vi "1big_with_d12.vi"() -> ()   [LabVIEW 2021]
panel:
  out "Waveform Graph":dbl[](graph)=[0.0, 0.0048018876, 0.018431017, 0.039760882, 0.067719858, 0.10129508, 0.13953534, 0.18155307, 0.2265255, 0.27369508, 0.32236922, 0.37191952, 0.42178034, 0.47144713, 0.52047418, 0.56847222, 0.61510569, 0.66008982, 0.70318758, 0.74420648, 0.78299539, 0.81944126, 0.8534659, 0.88502272, 0.91409368, 0.94068615, 0.96483002, 0.98657486, 1.0059872, 1.023148, 1.0381504, 1.0510971, 1.0620986, 1.0712715, 1.078736, 1.0846151, 1.0890327, 1.0921125, 1.0939767, 1.0947453, 1.0945349, 1.0934583, 1.0916234, 1.0891333, 1.0860856, 1.082572, 1.0786782, 1.074484, 1.0700627, 1.0654817, 1.0608022, 1.0560794, 1.0513626, 1.0466956, 1.0421167, 1.037659, 1.0333508, 1.0292157, 1.0252732, 1.0215385, 1.0180234, 1.014736, 1.0116817, 1.0088627, 1.006279, 1.0039284, 1.0018066, 0.99990777, 0.99822449, 0.99674827, 0.9954696, 0.99437817, 0.9934631, 0.99271305, 0.99211642, 0.99166149, 0.99133651, 0.99112985, 0.99103008, 0.99102605, 0.99110696, 0.99126246, 0.99148264, 0.99175812, 0.99208005, 0.99244014, 0.9928307, 0.99324459, 0.99367528, 0.99411683, 0.99456383, 0.99501148, 0.99545547, 0.99589204, 0.99631793, 0.99673032, 0.99712687, 0.99750563, 0.99786504, 0.99820391, 0.99852138, 0.99881687, 0.99909008, 0.99934096, 0.99956969, 0.99977659, 0.99996221, 1.0001272, 1.0002723, 1.0003985, 1.0005066, 1.0005977, 1.000673, 1.0007333, 1.0007799, 1.000814, 1.0008365, 1.0008486, 1.0008513, 1.0008457, 1.0008328, 1.0008135, 1.0007887, 1.0007593, 1.0007261, 1.0006897, 1.000651, 1.0006106, 1.000569, 1.0005267, 1.0004842, 1.000442, 1.0004004, 1.0003598, 1.0003203, 1.0002823, 1.0002459, 1.0002114, 1.0001787, 1.0001481, 1.0001195, 1.000093, 1.0000687, 1.0000464, 1.0000263, 1.0000081, 0.99999198, 0.99997772, 0.99996529, 0.99995459, 0.99994552, 0.999938, 0.99993191, 0.99992715, 0.99992361, 0.99992119, 0.99991979, 0.9999193, 0.99991963, 0.99992068, 0.99992235, 0.99992457, 0.99992724, 0.9999303, 0.99993367, 0.99993728, 0.99994108, 0.999945, 0.99994899, 0.99995302, 0.99995703, 0.99996099, 0.99996487, 0.99996864, 0.99997229, 0.99997578, 0.9999791, 0.99998225, 0.9999852, 0.99998796, 0.99999053, 0.99999289, 0.99999505, 0.99999701, 0.99999878, 1.0000004, 1.0000018, 1.000003, 1.000004, 1.0000049, 1.0000057, 1.0000063, 1.0000068, 1.0000072, 1.0000074, 1.0000076, 1.0000076, 1.0000076, 1.0000076, 1.0000074, 1.0000072]
  out "size(s)":i32[](array[numeric])=[603, 2]
  out "Signals 2":dbl=1.0000072
  out "Signals":dynamicdata(graph)=[{"t0"=timestamp(0 s since 1904-01-01), "dt"=1.0, "Y"=array[603 elements], "attributes"=variant("NI_ChannelName"=variant(string ""), "NI_ExpIsRelativeTime"=variant(bool FALSE), "NI_ExpStartTimeStamp"=variant(timestamp timestamp(0 s since 1904-01-01)), "NI_ExpTimeStamp"=variant(timestamp timestamp(0 s since 1904-01-01)), "NI_ExpXDimension"=variant(string ""))}, {"t0"=timestamp(0 s since 1904-01-01), "dt"=1.0, "Y"=[0.0, 0.0, 0.0, 0.0, 0.0, 0.0, 0.0, 0.0, 0.0, 0.0, 0.0, 0.0, 0.0, 0.0, 0.0, 0.0, 0.0, 0.0, 0.0, 0.0, 0.0, 0.0, 0.0, 0.0, 0.0, 0.0, 0.0, 0.0, 0.0, 0.0, 0.0, 0.0, 0.0, 0.0, 0.0, 0.0, 0.0, 0.0, 0.0, 0.0, 0.0, 0.0, 0.0, 0.0, 0.0, 0.0, 0.0, 0.0, 0.0, 0.0, 0.0, 0.0, 0.0, 0.0, 0.0, 0.0, 0.0, 0.0, 0.0, 0.0, 0.0, 0.0, 0.0, 0.0, 0.0, 0.0, 0.0, 0.0, 0.0, 0.0, 0.0, 0.0, 0.0, 0.0, 0.0, 0.0, 0.0, 0.0, 0.0, 0.0, 0.0, 0.0, 0.0, 0.0, 0.0, 0.0, 0.0, 0.0, 0.0, 0.0, 0.0, 0.0, 0.0, 0.0, 0.0, 0.0, 0.0, 0.0, 0.0, 0.0, 0.0, 0.0, 0.0, 0.0, 0.0, 0.0, 0.0, 0.0, 0.0, 0.0, 0.0, 0.0, 0.0, 0.0, 0.0, 0.0, 0.0, 0.0, 0.0, 0.0, 0.0, 0.0, 0.0, 0.0, 0.0, 0.0, 0.0, 0.0, 0.0, 0.0, 0.0, 0.0, 0.0, 0.0, 0.0, 0.0, 0.0, 0.0, 0.0, 0.0, 0.0, 0.0, 0.0, 0.0, 0.0, 0.0, 0.0, 0.0, 0.0, 0.0, 0.0, 0.0, 0.0, 0.0, 0.0, 0.0, 0.0, 0.0, 0.0, 0.0, 0.0, 0.0, 0.0, 0.0, 0.0, 0.0, 0.0, 0.0, 0.0, 0.0, 0.0, 0.0, 0.0, 0.0, 0.0, 0.0, 0.0, 0.0, 0.0, 0.0, 0.0, 0.0, 0.0, 0.0, 0.0, 0.0, 0.0, 0.0, 0.0, 0.0, 0.0, 0.0, 0.0, 0.0, 0.0, 0.0, 0.0, 0.0, 0.0, 0.0, 0.0, 0.0, 0.0, 0.0, 0.0, 0.0, 0.0, 0.0, 0.0, 0.0, 0.0, 0.0, 0.0, 0.0, 0.0, 0.0, 0.0, 0.0, 0.0, 0.0, 0.0, 0.0, 0.0, 0.0, 0.0, 0.0, 0.0, 0.0, 0.0, 0.0, 0.0, 0.0, 0.0, 0.0, 0.0, 0.0, 0.0, 0.0, 0.0, 0.0, 0.0, 0.0, 0.0, 0.0, 0.0, 0.0, 0.0, 0.0, 0.0, 0.0, 0.0, 0.0, 0.0, 0.0, 0.0, 0.0, 0.0, 0.0, 0.0, 0.0, 0.0, 0.0, 0.0, 0.0, 0.0, 0.0, 0.0, 0.0, 0.0, 0.0, 0.0, 0.0, 0.0, 0.0, 0.0, 0.0, 0.0, 0.0, 0.0, 0.0, 0.0, 0.0, 0.0, 0.0, 0.0, 0.0, 0.0, 0.0, 0.0, 0.0, 0.0, 0.0, 0.0, 0.0, 0.0, 0.0, 0.0, 0.0, 0.0, 0.0, 0.0, 0.0, 0.0, 0.0, 0.0, 0.0, 0.0, 0.0, 0.0, 0.0, 0.0, 0.0, 0.0, 0.0, 0.0, 0.0, 0.0, 0.0, 0.0, 0.0, 0.0, 0.0, 0.0, 0.0, 0.0, 0.0, 0.0, 0.0, 0.0, 0.0, 0.0, 0.0, 0.0, 0.0, 0.0, 0.0, 0.0, 0.0, 0.0, 0.0, 0.0, 0.0, 0.0, 0.0, 0.0, 0.0, 0.0, 0.0, 0.0, 0.0, 0.0, 0.0, 0.0, 0.0, 0.0, 0.0, 0.0, 0.0, 0.0, 0.0, 0.0, 0.0, 0.0, 0.0, 0.0, 0.0, 0.0, 0.0, 0.0, 0.0, 0.0, 0.0, 0.0, 0.0, 0.0, 0.0, 0.0, 0.0, 0.0, 0.0, 0.0, 0.0, 0.0, 0.0, 0.0, 0.0, 0.0, 0.0, 0.0, 0.0, 0.0, 0.0, 0.0, 0.0, 0.0, 0.0, 0.0, 0.0, 0.0, 0.0, 0.0, 0.0, 0.0, 0.0, 0.0, 0.0, 0.0, 0.0, 0.0, 0.0, 0.0, 0.0, 0.0, 0.0, 0.0, 0.0, 0.0, 0.0, 0.0, 0.0, 0.0, 0.0, 0.0, 0.0, 0.0, 0.0, 0.0, 0.0, 0.0, 0.0, 0.0, 0.0, 0.0, 0.0, 0.0, 0.0, 0.0, 0.0, 0.0, 0.0, 0.0, 0.0, 0.0, 0.0, 0.0, 0.0, 0.0, 0.0, 0.0, 0.0, 0.0, 0.0, 0.0, 0.0, 0.0, 0.0, 0.0, 0.0, 0.0, 0.0, 0.0, 0.0, 0.0, 0.0, 0.0, 0.0, 0.0, 0.0, 0.0, 0.0, 0.0, 0.0, 0.0, 0.0, 0.0, 0.0, 0.0, 0.0, 0.0, 0.0, 0.0, 0.0, 0.0, 0.0, 0.0, 0.0, 0.0, 0.0, 0.0, 0.0, 0.0, 0.0, 0.0, 0.0, 0.0, 0.0, 0.0, 0.0, 0.0, 0.0, 0.0, 0.0, 0.0, 0.0, 0.0, 0.0, 0.0, 0.0, 0.0, 0.0, 0.0, 0.0, 0.0, 0.0, 0.0, 0.0, 0.0, 0.0, 0.0, 0.0, 0.0, 0.0, 0.0, 0.0, 0.0, 0.0, 0.0, 0.0, 0.0, 0.0, 0.0, 0.0, 0.0, 0.0, 0.0, 0.0, 0.0, 0.0, 0.0, 0.0, 0.0, 0.0, 0.0, 0.0, 0.0, 0.0, 0.0, 0.0, 0.0, 0.0, 0.0, 0.0, 0.0, 0.0, 0.0, 0.0, 0.0, 0.0, 0.0, 0.0, 0.0, 0.0, 0.0, 0.0, 0.0, 0.0, 0.0, 0.0, 0.0, 0.0, 0.0, 0.0, 0.0, 0.0, 0.0, 0.0, 0.0, 0.0, 0.0, 0.0, 0.0, 0.0, 0.0, 0.0, 0.0, 0.0, 0.0, 0.0, 0.0, 0.0, 0.0, 0.0, 0.0, 0.0, 0.0, 0.0, 0.0, 0.0, 0.0, 0.0, 0.0, 0.0, 0.0], "attributes"=variant("NI_ChannelName"=variant(string ""), "NI_ExpIsRelativeTime"=variant(bool FALSE), "NI_ExpStartTimeStamp"=variant(timestamp timestamp(0 s since 1904-01-01)), "NI_ExpTimeStamp"=variant(timestamp timestamp(0 s since 1904-01-01)), "NI_ExpXDimension"=variant(string ""))}]
  in  "Filename":path=path "E:/Programando Linx/Clase 1/data12.lvm"
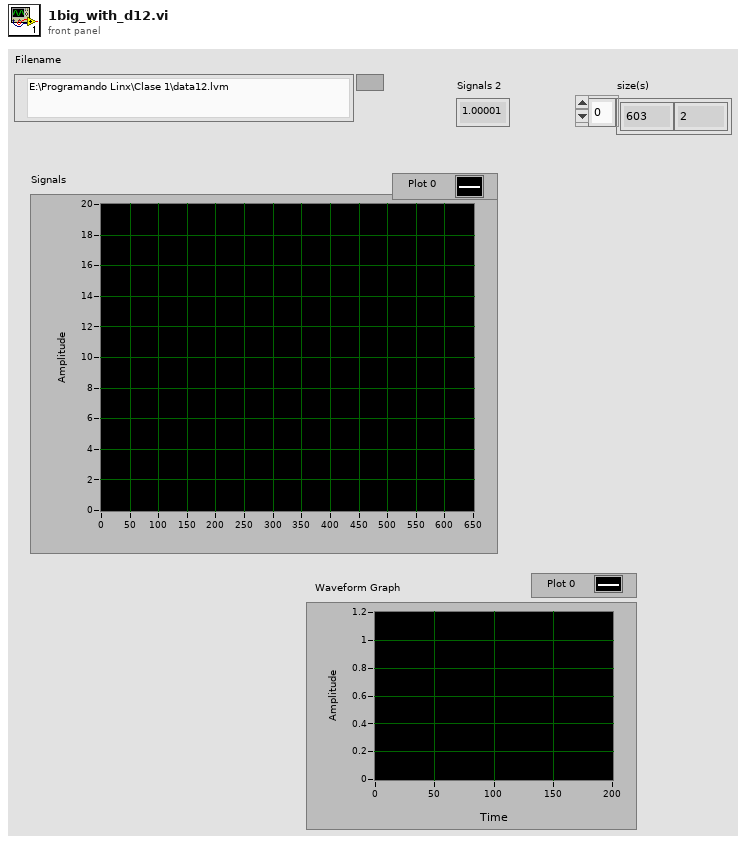
[diagram p1: front panel]
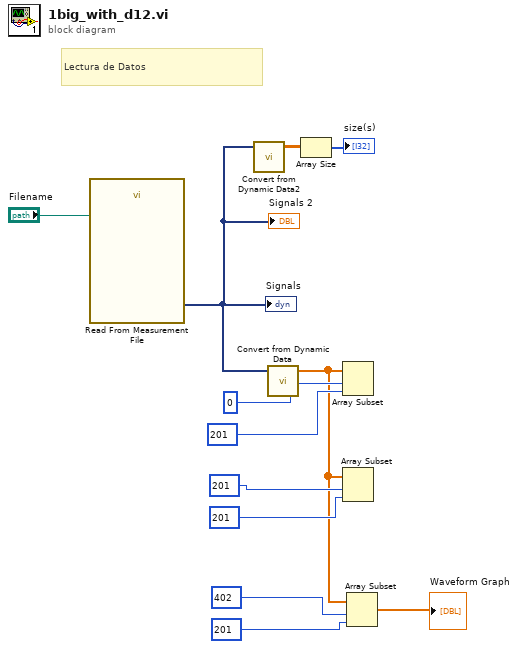
[diagram p0: block diagram]
diagram:
  # "Lectura de Datos"
  n1 = call "Read From Measurement File"("Filename"="Filename") -> ("Signals"=w9:dynamicdata)  [unwired: 5 in, 5 out]
  "Signals" <- w9
  "Signals 2" <- w9
  n2 = call "Convert from Dynamic Data2"("Dynamic Data Type"=w9) -> ("Array"=w11:dbl[][])  [unwired: 3 in]
  n3 = call "Convert from Dynamic Data"("Dynamic Data Type"=w9) -> ("Array"=w4:dbl[])  [unwired: 3 in]
  n4 = Array Size(array=w11) -> (size(s)=→"size(s)":i32[])
  n5 = Array Subset(array=w4, index=0, length=201) -> ()  [unwired: 1 out]
  n6 = Array Subset(array=w4, index=201, length=201) -> ()  [unwired: 1 out]
  n7 = Array Subset(array=w4, index=402, length=201) -> (→"Waveform Graph":dbl[])
